vi "FCA create tdms file.vi"(10 "Filename prefix":string, 11 "Folder path":path) -> (0 "error out":errorcluster, 3 "Refnum out":refnum<k34>)   [LabVIEW 2020]
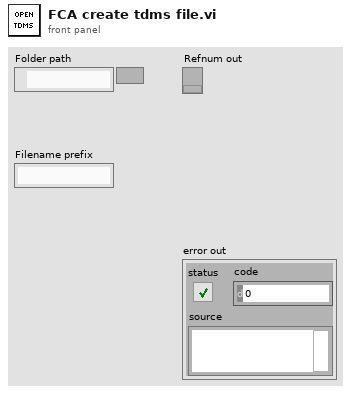
[diagram p1: front panel]
types:
  T1 = enum16{"open", "open or create", "create or replace", "create", "open (read-only)"}
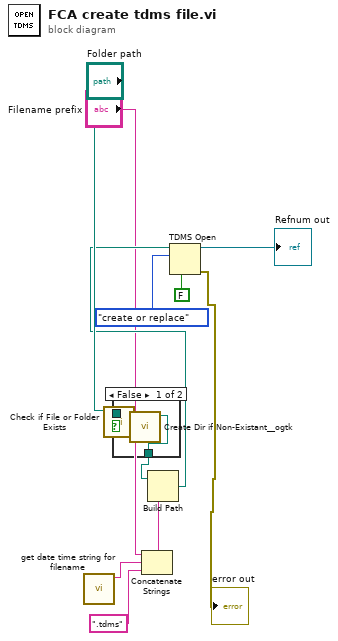
[diagram p0: block diagram]
diagram:
  n1 = call "get date time string for filename.vi"() -> ("time string"=w5:string)  [unwired: 11 in]
  n2 = call <vilib>:"Check if File or Folder Exists.vi"("path"="Folder path") -> ("file or folder exists?"=w10:bool, "dup path"=w12:path)  [unwired: 8 in, 1 out]
  n3 = case shown="False" w10 {
    tunnel: [w14 w16] -> w13
    tunnel: w12 -> [w15 w16]
    frame False {
      n4 = call <userlib>:"Create Dir if Non-Existant__ogtk.vi"("Directory Path"=w15) -> ("dup Directory Path"=w14:path)  [unwired: 8 in, 2 out]
    }
    frame True {
    }
  }
  n5 = Concatenate Strings("Filename prefix", w5, ".tdms" ("string")) -> (w7:string)
  n6 = Build Path(base path=w13, name or relative path=w7) -> (appended path=w8:path)
  n7 = TDMS Open(6:FALSE ("disable buffering (T)"), 10:T1."create or replace" ("operation"), 11:w8) -> (0:→"error out":errorcluster, 3:→"Refnum out":refnum<k34>)  [unwired: 4 in]
